vi "Model--Remove from Group.vi"(8 "error in":errorcluster, 11 "Selector in":refnum<class "Selector.lvclass">) -> (0 "error out":errorcluster, 2 "Name":string, 3 "Selector out":refnum<class "Selector.lvclass">)   [LabVIEW 2019, in "Selector.lvclass"]
uses:
  Selector.lvclass
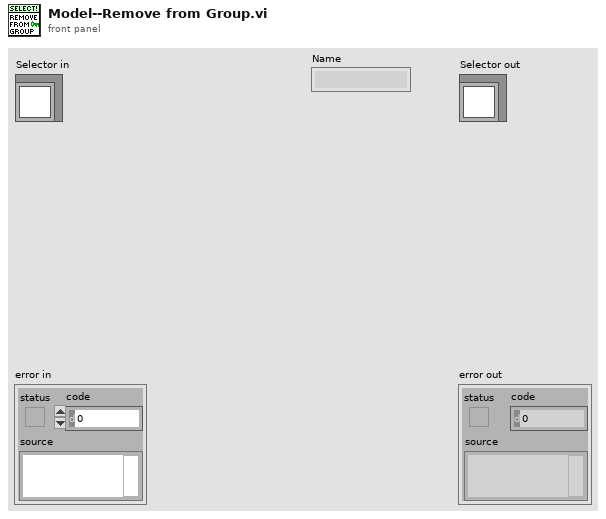
[diagram p1: front panel]
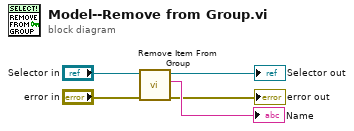
[diagram p0: block diagram]
diagram:
  n1 = call-dynamic "Remove Item From Group.vi"("error in (no error)"="error in", "Selector in"="Selector in") -> ("error out"=→"error out":errorcluster, "Name"=→"Name":string, "Selector out"=→"Selector out":refnum<class "Selector.lvclass">)  [unwired: 7 in]
